vi "ModelParameterValueUpdateFromFile.vi"(9 "Target":string, 10 "parameter_files":string[](array[string])) -> (0 "error out":errorcluster, 1 "Target out":string, 2 "parameter_files out":string[](array[string]))   [LabVIEW 2015, in "ni-veristand-steps-runtime-lib.lvlib"]
uses:
  ni-veristand-steps-runtime-lib.lvlib
  NationalInstruments.VeriStand.ClientAPI
  NationalInstruments.VeriStand
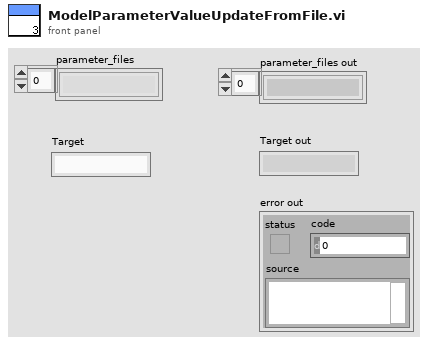
[diagram p1: front panel]
types:
  T1 = typedef "ni-veristand-steps-runtime-lib.lvlib/VeriStand dotNet References.ctl" = cluster{"Project Ref":refnum<k24>, "ModelManager":T2, "AlarmManager":T3, "ChannelFault":T4, "WorkspaceManager":T5}
  T2 = typedef "NI_VS ModelManager ExecutionAPI.lvlib/ModelManagerAPI.ctl" = refnum<k24>
  T3 = typedef "NI_VS AlarmManager ExecutionAPI.lvlib/AlarmManagerAPI.ctl" = refnum<k24>
  T4 = typedef "NI_VS ChannelFault ExecutionAPI.lvlib/ChannelFaultAPI.ctl" = refnum<k24>
  T5 = typedef "NI_VS Workspace ExecutionAPI.lvlib/WorkspaceAPI.ctl" = refnum<k24>
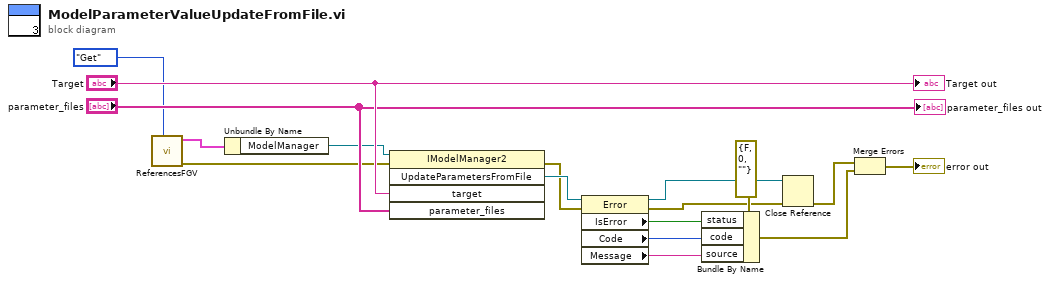
[diagram p0: block diagram]
diagram:
  n1 = call "ReferencesFGV.vi"("Get/Set"=enum16{"Get", "Set"}."Get") -> ("error out"=w4:errorcluster, "VeriStand dotNET Refs out"=w2:T1)  [unwired: 9 in]
  n2 = Unbundle By Name(w2) -> ("ModelManager"=w3:T2)
  n3 = invoke class="IModelManager2" method="UpdateParametersFromFile"(reference=w3, error in=w4, "target"="Target", "parameter_files"="parameter_files") -> (error out=w10:errorcluster, "UpdateParametersFromFile"=w16:refnum<k24>)  [unwired: 1 in, 3 out]
  n4 = property class="Error"(reference=w16, error in=w10) -> (reference out=w8:refnum<k24>, error out=w9:errorcluster, "IsError"=w12:bool, "Code"=w13:u32, "Message"=w14:string)
  n5 = Bundle By Name(cluster=errorcluster {"status"=FALSE, "code"=0, "source"=""} ("error in (no error)"), "status"=w12, "code"=w13, "source"=w14) -> (w6:errorcluster)
  n6 = Close Reference(reference=w8, error in (no error)=w9) -> (error out=w7:errorcluster)
  n7 = Merge Errors(w7, w6) -> (→"error out":errorcluster)
  "Target out" <- "Target"
  "parameter_files out" <- "parameter_files"
